vi "Set Parameter Bit Encoding.vi"(5 "signed?":bool, 7 "encoding":T1, 8 "error in":errorcluster, 9 "number of bits":i32, 10 "start bit":i32, 11 "parameter ref in":T2 format="%.0x") -> (0 "error out":errorcluster, 3 "parameter ref out":T2 format="%.0x")   [LabVIEW 2020, in "ARINC 429 Scripting.lvlib"]
uses:
  ARINC 429 Scripting.lvlib
  <vilib>/NI VeriStand/Custom Device API/Custom Device Item Ref.ctl
  <vilib>/NI/NI VeriStand Encoding and Decoding/Encoding.ctl
  Constants.vi
  <vilib>/NI VeriStand/Custom Device API/Set Item Property (U16).vi
  <vilib>/NI VeriStand/Custom Device API/Set Item Property (I32).vi
  <vilib>/NI VeriStand/Custom Device API/Set Item Property (Boolean).vi
  <vilib>/NI VeriStand/Custom Device API/Custom Device API.lvlib
  <vilib>/NI/NI VeriStand Encoding and Decoding/Encoding and Decoding.lvlib
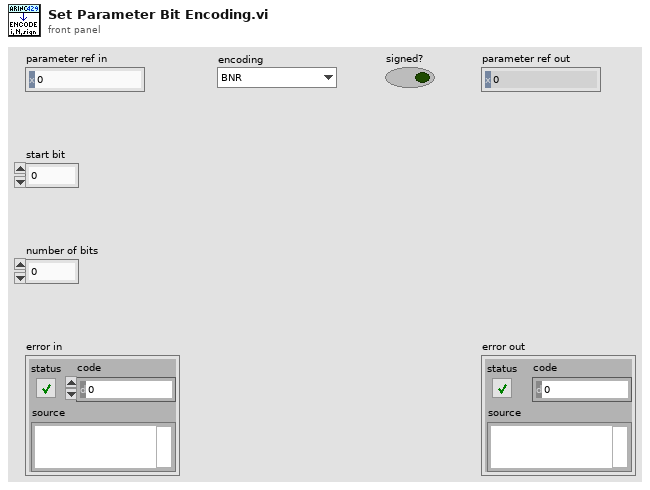
[diagram p1: front panel]
types:
  T1 = typedef "Encoding and Decoding.lvlib/Encoding.ctl" = enum16{"BNR", "BCD", "Discrete"}
  T2 = typedef "Custom Device API.lvlib/Custom Device Item Ref.ctl" = u64
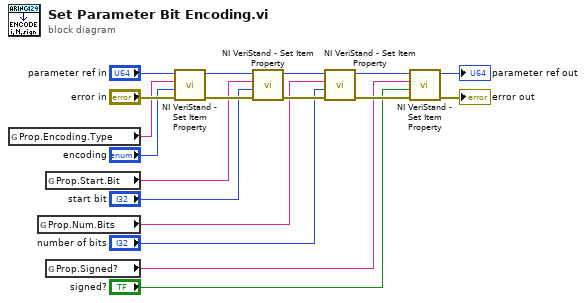
[diagram p0: block diagram]
diagram:
  n1 = global read "Constants.vi" "Prop.Encoding.Type"() -> (w7:string)
  n2 = global read "Constants.vi" "Prop.Num.Bits"() -> (w5:string)
  n3 = global read "Constants.vi" "Prop.Start.Bit"() -> (w6:string)
  n4 = global read "Constants.vi" "Prop.Signed?"() -> (w8:string)
  n5 = call-poly <vilib>:"NI VeriStand - Set Item Property.vi"("error in (no error)"="error in", "Value"="encoding", "Property Name"=w7, "Item Ref in"="parameter ref in") -> ("error out"=w13:errorcluster, "Item Ref out"=w14:T2)  [unwired: 5 in, 1 out]
  n6 = call-poly <vilib>:"NI VeriStand - Set Item Property.vi"("error in (no error)"=w13, "Value"="start bit", "Property Name"=w6, "Item Ref in"=w14) -> ("error out"=w11:errorcluster, "Item Ref out"=w12:T2)  [unwired: 5 in, 1 out]
  n7 = call-poly <vilib>:"NI VeriStand - Set Item Property.vi"("error in (no error)"=w11, "Value"="number of bits", "Property Name"=w5, "Item Ref in"=w12) -> ("error out"=w9:errorcluster, "Item Ref out"=w10:T2)  [unwired: 5 in, 1 out]
  n8 = call-poly <vilib>:"NI VeriStand - Set Item Property.vi"("error in (no error)"=w9, "Value"="signed?", "Property Name"=w8, "Item Ref in"=w10) -> ("error out"=→"error out":errorcluster, "Item Ref out"=→"parameter ref out":T2)  [unwired: 5 in, 1 out]
